vi "rrtOffensiveWhile.vi"(6 "AttackerAvoidArea":bool=TRUE, 8 "error in (no error)":errorcluster, 9 "Line?":bool=TRUE, 10 "Volta ao redor\nda área?":bool, 11 "GameReference in":refnum<data-value>) -> (0 "error out":errorcluster)   [LabVIEW 2020, in "Game.lvclass"]
uses:
  Game.lvclass
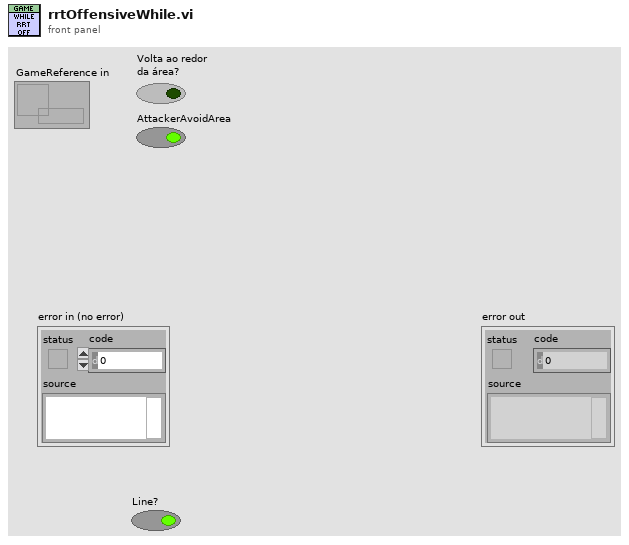
[diagram p1: front panel]
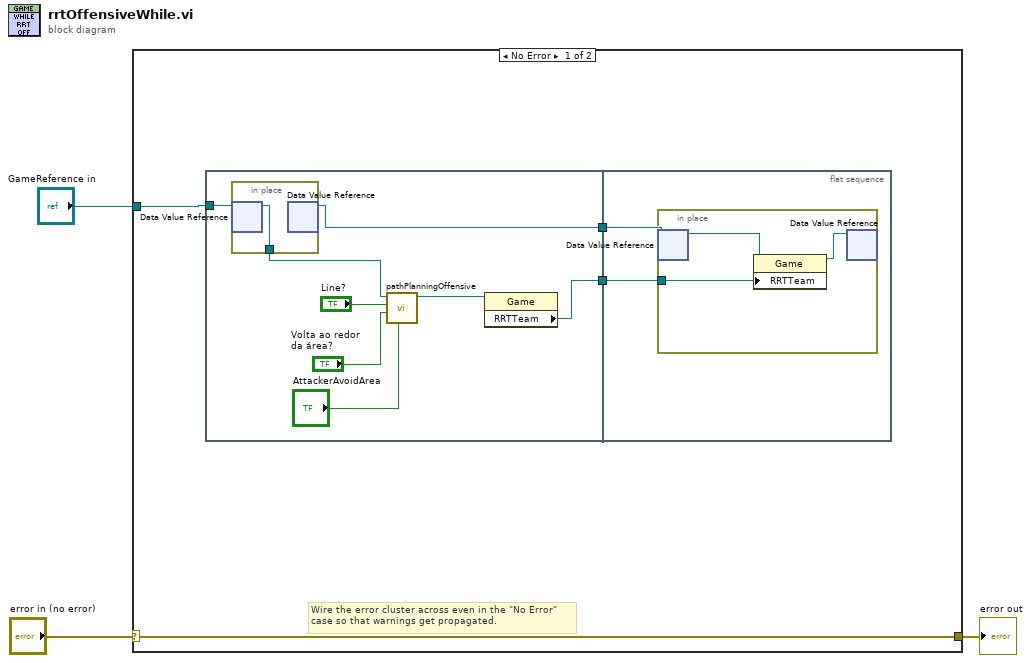
[diagram p0: block diagram]
diagram:
  n1 = case shown="No Error" "error in (no error)" {
    selector: "error in (no error)" -> [w7 w22]
    tunnel: [w7 w22] -> w2
    tunnel: "GameReference in" -> [w6 _]
    frame No Error {
      # "Wire the error cluster across even in the \"No Error\"\ncase so that warnings get propagated."
      n2 = flat-sequence {
        tunnel: w6 -> [w15]
        tunnel: [w14] -> w5
        tunnel: [w13] -> w4
        tunnel: w5 -> [w18]
        tunnel: w4 -> [w17]
        frame #0 {
          n3 = in-place {
            in-place-border: [w16] -> w10
            n4 = in-place-dvr #1(w15) -> (w16:refnum<class "Game.lvclass">)  [unwired: 1 out]
            n5 = in-place-dvr #1() -> (w13:refnum<data-value>)  [unwired: 1 in, 1 out]
          }
          n6 = call-dynamic "pathPlanningOffensive.vi"("AttackerAvoidArea"="AttackerAvoidArea", "Volta ao redor\nda área?"="Volta ao redor\nda área?", "Line?"="Line?", "Game in"=w10) -> ("Game out"=w12:refnum<class "Game.lvclass">)  [unwired: 6 in, 1 out]
          n7 = property class="Game"(reference=w12) -> ("RRTTeam"=w14:refnum<class "Ally.lvclass">)  [unwired: 1 in, 2 out]
        }
        frame #1 {
          n8 = in-place {
            in-place-border: w18 -> [w21]
            n9 = in-place-dvr #2(w17) -> (w19:refnum<class "Game.lvclass">)  [unwired: 1 out]
            n10 = property class="Game"(reference=w19, "RRTTeam"=w21) -> (reference out=w20:refnum<class "Game.lvclass">)  [unwired: 1 in, 1 out]
            n11 = in-place-dvr #2(w20) -> ()  [unwired: 2 out]
          }
        }
      }
    }
    frame Error {
    }
  }
  "error out" <- w2
